vi "Input Multiple Build String Array.vi"(7 "Input Array":u8[][](array[numeric])) -> (8 "String Array":string[][](array[string]))   [LabVIEW 2010]
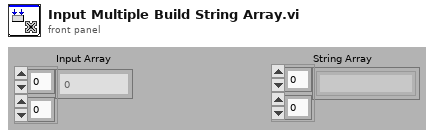
[diagram p1: front panel]
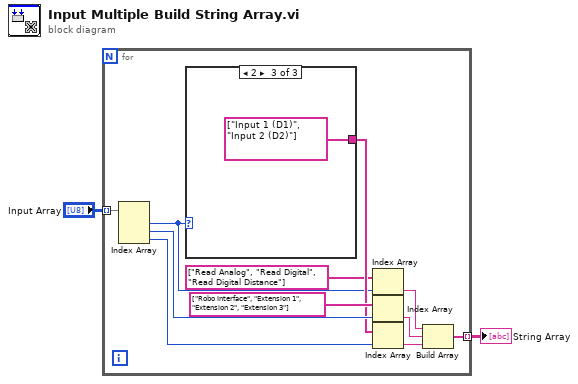
[diagram p0: block diagram]
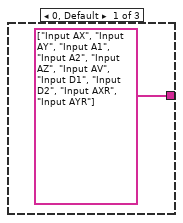
[diagram p2: hidden frame]
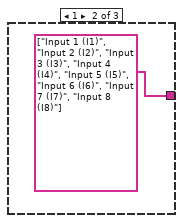
[diagram p3: hidden frame]
diagram:
  n1 = for {
    tunnel: "Input Array" -> [w13] mode=indexing
    tunnel: [w6] -> w1 mode=indexing
    n2 = Index Array(array=w13) -> (element #1=w3:u8, element #2=w11:u8, element #3=w10:u8)  [unwired: 3 in]
    n3 = case shown="2" w3 {
      tunnel: [string[] ["Input AX", "Input AY", "Input A1", "Input A2", "Input AZ", "Input AV", "Input D1", "Input D2", "Input AXR", "Input AYR"] string[] ["Input 1 (I1)", "Input 2 (I2)", "Input 3 (I3)", "Input 4 (I4)", "Input 5 (I5)", "Input 6 (I6)", "Input 7 (I7)", "Input 8 (I8)"] string[] ["Input 1 (D1)", "Input 2 (D2)"]] -> w5
      frame 0, Default {
      }
      frame 1 {
      }
      frame 2 {
      }
    }
    n4 = Index Array(array=string[] ["Read Analog", "Read Digital", "Read Digital Distance"], index=w3) -> (element=w9:string)
    n5 = Index Array(array=string[] ["Robo Interface", "Extension 1", "Extension 2", "Extension 3"] ("Strings [] 2"), index=w11) -> (element=w8:string)
    n6 = Index Array(array=w5, index=w10) -> (element=w7:string)
    n7 = Build Array(w9, w8, w7) -> (w6:string[])
  }
  "String Array" <- w1
